vi "Compensa attriti.vi"(7 "BANCO":i32, 8 "Procedura abilitata?":bool, 9 "C[Nm] in":dbl format="%#_13g", 10 "rpm":dbl format="%#_13g", 11 "Cluster INFO":T1={"Scelta wattmetro"={"Wattmetro"=enum."No Selection"}, "SET RPM"=0.0, "SET TEMP"=0.0, "Array banchi"=[{"Nome"="Elettropompa", "Tors. scala1"=0, "Tors. scala2"=0, "rpm"=0, "TAMB"=0, "Indici Temperature"=[0, 1], "Indice freno"=1, "alimentatore trifase"=0, "alimentatore monofase"=0, "alimentatore dc arm"=0, "alimentatore dc ecc"=0, "alimentatore dc mp"=0}, {"Nome"="Sommersa", "Tors. scala1"=0, "Tors. scala2"=0, "rpm"=0, "TAMB"=1, "Indici Temperature"=[0, 1], "Indice freno"=0, "alimentatore trifase"=0, "alimentatore monofase"=0, "alimentatore dc arm"=0, "alimentatore dc ecc"=0, "alimentatore dc mp"=0}], "Array valvole linee avvio/fermata"=[], "banco selezionato"=0, "Nomi valvole prop sistema"=[], "canale-- sensore"=[], "Attriti B1"=[], "Attriti B2"=[], "Collegamento elettrico"={"ALIMENTAZIONE ELETTRICA"=enum."AC TRIFASE", "ID"=0, "#rami freddo\\eq term resmeter"=0, "#rami riscaldamento resmeter"=0, "#rami freddo\\eq term resistomat"=0, "#rami riscaldamento resistomat"=0, "CALCOLI"=enum."AC TRIFASE"}, "lingua"=0, "Costanti collaudo"={"P [bar]"=0.0, "T amb. [°C]"=0.0, "Umidità [%]"=0.0, "T acqua [°C] 2"=0.0}, "OPZIONI MISURE RES"={"MISURA A FREDDO"=enum."RESISTOMAT", "MISURA EQ. TERMICO"=enum."RESISTOMAT", "MISURA DT PROVA IN CORSO"=enum."RESISTOMAT - CON FERMATE", "MISURE PRIMA E DOPO"=enum."RESISTOMAT", "STRUMENTI PRESENTI"=enum."NESSUNO"}, "Dati targa motore"={"Vnom"=0.0, "Fnom"=0.0, "Inom"=0.0, "Cnom"=0.0, "Npoli"=0.0, "Scorta 1"=0.0, "Scorta 2"=0.0, "Scorta 3"=0.0}}) -> (3 "C[Nm] out":dbl)   [LabVIEW 2019]
uses:
  TypeDef/Cluster INFO.ctl
  TypeDef/WT SELECTION.ctl
  TypeDef/Definizione linea.ctl
  TypeDef/Collegamenti_elettrici.ctl
  TypeDef/Control Calcoli.ctl
  <vilib>/gmath/NI_Gmath.lvlib
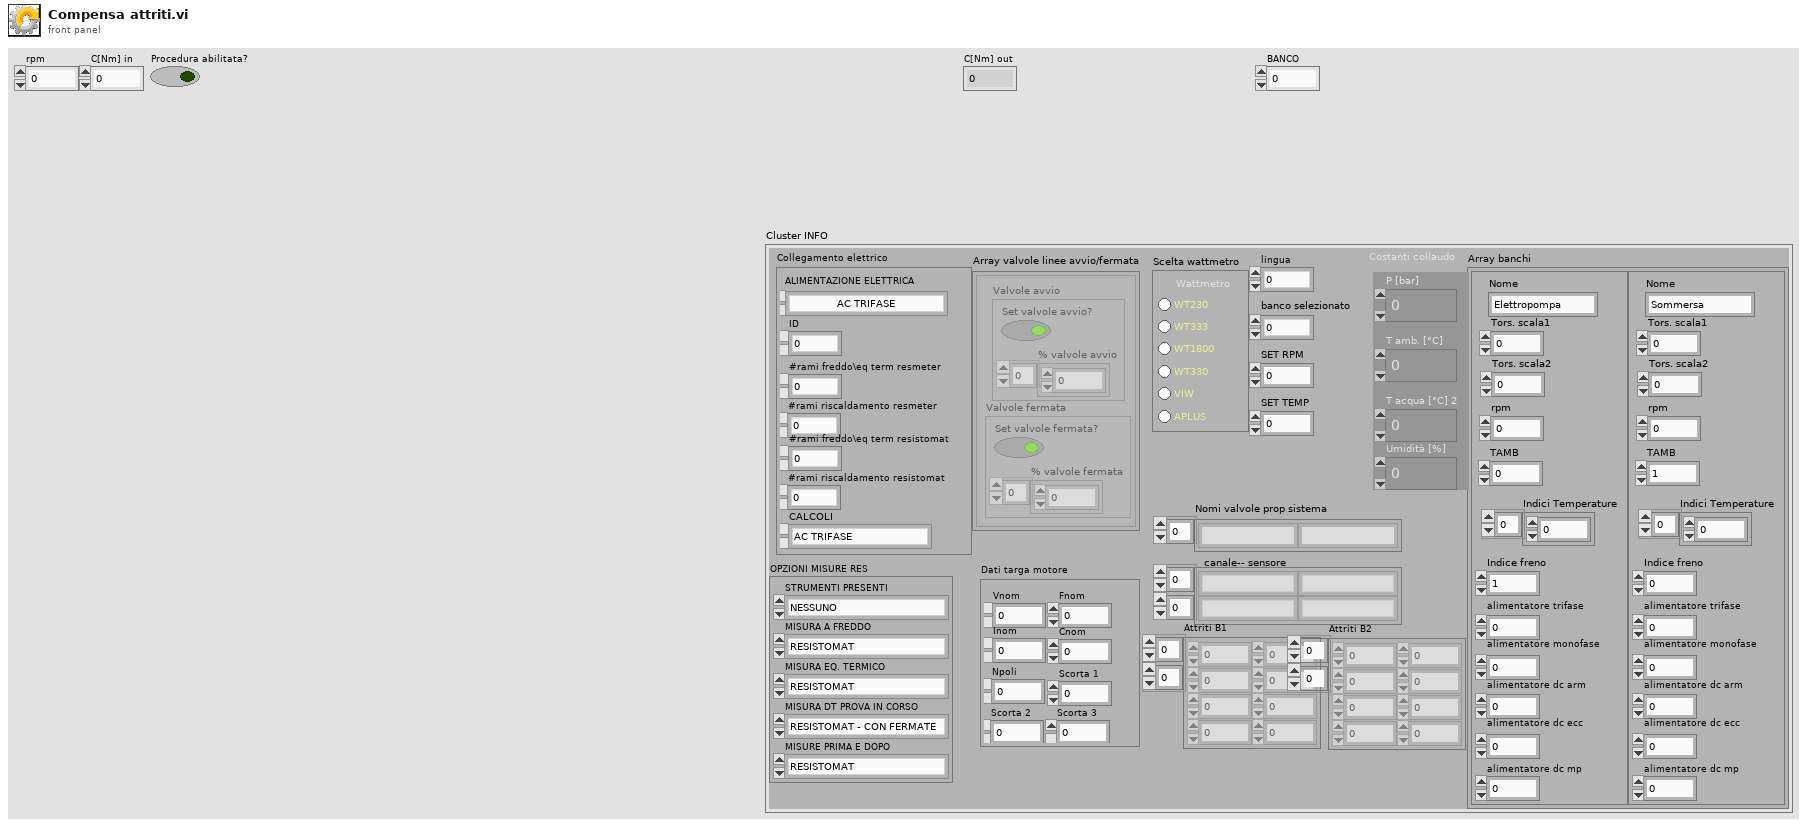
[diagram p1: front panel]
types:
  T1 = typedef "Cluster INFO.ctl" = cluster{"Scelta wattmetro":cluster{"Wattmetro":T2}, "SET RPM":dbl, "SET TEMP":dbl, "Array banchi":T3[], "Array valvole linee avvio/fermata":cluster{"Valvole avvio":cluster{"Set valvole avvio?":bool, "% valvole avvio":dbl[]}, "Valvole fermata":cluster{"Set valvole fermata?":bool, "% valvole fermata":dbl[]}}[], "banco selezionato":i8, "Nomi valvole prop sistema":string[], "canale-- sensore":string[][], "Attriti B1":dbl[][], "Attriti B2":dbl[][], "Collegamento elettrico":cluster{"ALIMENTAZIONE ELETTRICA":T4, "ID":i16, "#rami freddo\\eq term resmeter":i16, "#rami riscaldamento resmeter":i16, "#rami freddo\\eq term resistomat":i16, "#rami riscaldamento resistomat":i16, "CALCOLI":T5}, "lingua":i16, "Costanti collaudo":cluster{"P [bar]":dbl, "T amb. [°C]":dbl, "Umidità [%]":dbl, "T acqua [°C] 2":dbl}, "OPZIONI MISURE RES":cluster{"MISURA A FREDDO":enum16{"NESSUNO", "RESISTOMAT", "RES METER", "ENTRAMBI"}, "MISURA EQ. TERMICO":enum16{"NESSUNO", "RESISTOMAT", "RES METER", "ENTRAMBI"}, "MISURA DT PROVA IN CORSO":enum16{"NESSUNO", "RESISTOMAT - CON FERMATE", "RES METER - CON FERMATE", "RES METER - CONTINUO"}, "MISURE PRIMA E DOPO":enum16{"NESSUNO", "RESISTOMAT", "RES METER"}, "STRUMENTI PRESENTI":enum16{"NESSUNO", "RESISTOMAT", "RES METER", "ENTRAMBI"}}, "Dati targa motore":cluster{"Vnom":dbl, "Fnom":dbl, "Inom":dbl, "Cnom":dbl, "Npoli":dbl, "Scorta 1":dbl, "Scorta 2":dbl, "Scorta 3":dbl}}
  T2 = typedef "WT SELECTION.ctl" = enum32{"No Selection", "WT230", "WT333", "WT1800", "WT330", "VIW", "APLUS"}
  T3 = typedef "Definizione linea.ctl" = cluster{"Nome":string, "Tors. scala1":i32, "Tors. scala2":i32, "rpm":i32, "TAMB":i32, "Indici Temperature":i16[], "Indice freno":i16, "alimentatore trifase":i16, "alimentatore monofase":i16, "alimentatore dc arm":i16, "alimentatore dc ecc":i16, "alimentatore dc mp":i16}
  T4 = typedef "Collegamenti_elettrici.ctl" = enum16{"AC TRIFASE", "AC TRIFASE + FRENO", "AC MONOFASE", "DC CON ECCITAZIONE", "DC CON ECCITAZIONE + FRENO", "DC NO ECCITAZIONE", "DC NO ECCITAZIONE + FRENO", "FRENO TRASC + AFE", "SOLO FRENO", "CARICO RESISTIVO", "GENERICO", "SOLO ACQUISITORE", "SCORTA 4", "SCORTA 5", "SCORTA 6"}
  T5 = typedef "Control Calcoli.ctl" = enum16{"AC TRIFASE", "AC MONOFASE", "DC ECCITAZIONE", "DC NO ECCITAZIONE", "POMPA TRIFASE", "POMPA MONOFASE", "GENERICO", "TRASFORMATORE", "ALTERNATORE TRASCINATO", "GRUPPO ELETTROGENO"}
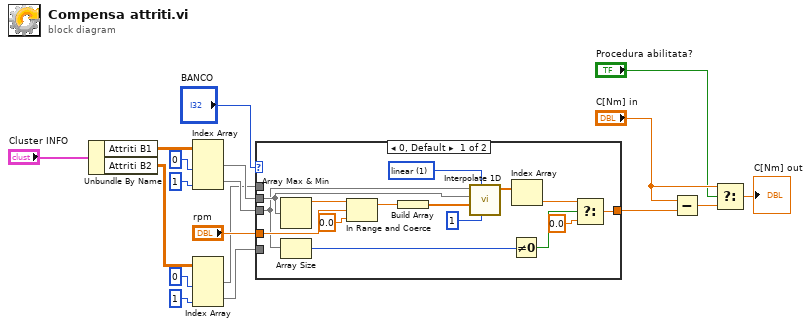
[diagram p0: block diagram]
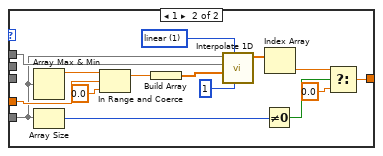
[diagram p2: hidden frame]
diagram:
  n1 = Unbundle By Name("Cluster INFO") -> ("Attriti B1"=w17:dbl[][], "Attriti B2"=w12:dbl[][])
  n2 = Index Array(array=w17, index (col) #1=0 ("disabled index (col)"), index (col) #2=1 ("index (col)")) -> (element #1=w11:dbl[], element #2=w10:dbl[])  [unwired: 2 in]
  n3 = Index Array(array=w12, index (col) #1=0 ("disabled index (col)"), index (col) #2=1 ("index (col)")) -> (element #1=w7:dbl[], element #2=w6:dbl[])  [unwired: 2 in]
  n4 = case shown="0, Default" "BANCO" {
    tunnel: w11 -> [w25 _]
    tunnel: w10 -> [w24 _]
    tunnel: [w20 w34] -> w8
    tunnel: "rpm" -> [w29 w41]
    tunnel: w7 -> [_ w40]
    tunnel: w6 -> [_ w37]
    frame 0, Default {
      w33 = 1 items=["nearest", "linear", "spline", "cubic Hermite", "Lagrange"] ("method")
      n5 = Array Max & Min(array=w25) -> (max value=w26:dbl)  [unwired: 3 out]
      n6 = Array Size(array=w24) -> (size(s)=w23:i32)
      n7 = In Range and Coerce(upper limit=w26, x=w29, lower limit=0.0) -> (coerced(x)=w28:dbl)  [unwired: 1 out]
      n8 = Build Array(w28) -> (w30:dbl[])
      n9 = call <vilib>:"Interpolate 1D.vi"("ntimes"=1, "method"=w33, "xi"=w30, "X"=w25, "Y"=w24) -> ("yi"=w31:dbl[])  [unwired: 4 in, 2 out]
      n10 = Not Equal To 0?(x=w23) -> (x != 0?=w22:bool)
      n11 = Index Array(array=w31) -> (element=w21:dbl)  [unwired: 1 in]
      n12 = Select(t=w21, s=w22, f=0.0) -> (s? t:f=w20:dbl)
    }
    frame 1 {
      w48 = 1 items=["nearest", "linear", "spline", "cubic Hermite", "Lagrange"] ("method")
      n13 = Array Max & Min(array=w37) -> (max value=w43:dbl)  [unwired: 3 out]
      n14 = Array Size(array=w37) -> (size(s)=w39:i32)
      n15 = In Range and Coerce(upper limit=w43, x=w41, lower limit=0.0) -> (coerced(x)=w45:dbl)  [unwired: 1 out]
      n16 = Build Array(w45) -> (w42:dbl[])
      n17 = call <vilib>:"Interpolate 1D.vi"("ntimes"=1, "method"=w48, "xi"=w42, "X"=w40, "Y"=w37) -> ("yi"=w46:dbl[])  [unwired: 4 in, 2 out]
      n18 = Not Equal To 0?(x=w39) -> (x != 0?=w36:bool)
      n19 = Index Array(array=w46) -> (element=w35:dbl)  [unwired: 1 in]
      n20 = Select(t=w35, s=w36, f=0.0) -> (s? t:f=w34:dbl)
    }
  }
  n21 = Subtract(x="C[Nm] in", y=w8) -> (x-y=w5:dbl)
  n22 = Select(t="C[Nm] in", s="Procedura abilitata?", f=w5) -> (s? t:f=→"C[Nm] out":dbl)
